vi "Write record log.vi"(4 "Year":i32, 6 "Month":i32, 7 "Instances in":T2[](array[typedef]), 8 "Error In":errorcluster, 11 "refnum":T1) -> (0 "Error Out":errorcluster, 3 "refnum out":T1)   [LabVIEW 2015]
uses:
  Home/Undelivered instance.ctl
  <vilib>/Utility/config.llb/Config Data RefNum.ctl
  <vilib>/Utility/config.llb/Read Key (Path).vi
  <vilib>/Utility/file.llb/Write Delimited Spreadsheet (string).vi
  <vilib>/Utility/config.llb/NI_LVConfig.lvlib
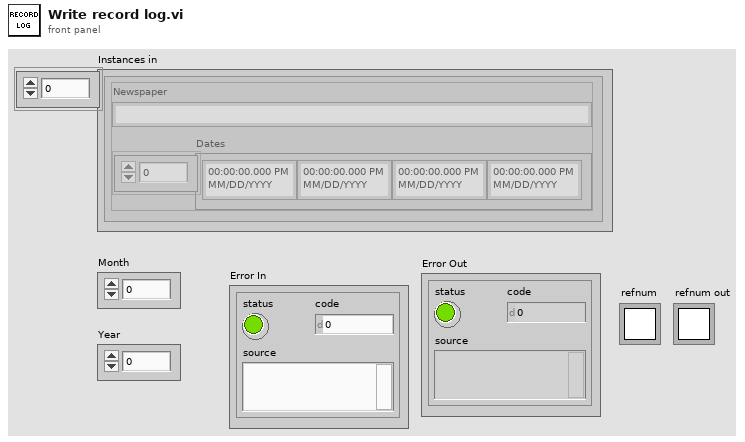
[diagram p1: front panel]
types:
  T1 = typedef "NI_LVConfig.lvlib/Config Data RefNum.ctl" = refnum<k1>
  T2 = typedef "Undelivered instance.ctl" = cluster{"Dates":timestamp[], "Newspaper":string}
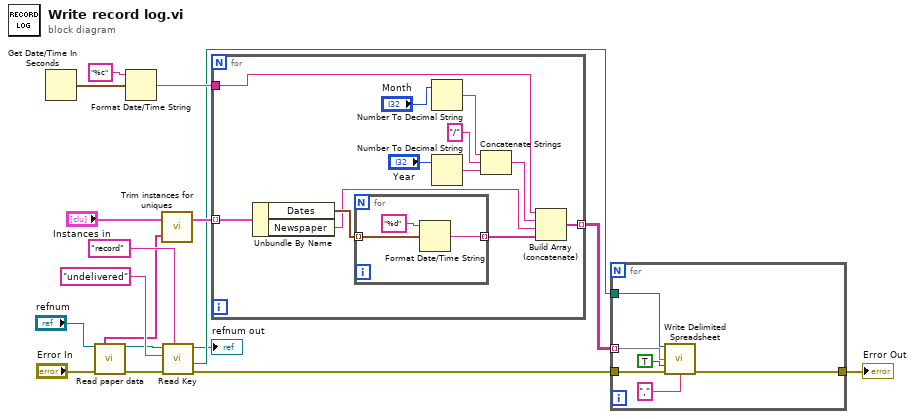
[diagram p0: block diagram]
diagram:
  n1 = Get Date/Time In Seconds() -> (seconds since 1Jan1904=w16:timestamp)
  n2 = call "Read paper data.vi"("Refnum in"="refnum", "error in (no error)"="Error In") -> ("Names"=w1:string[], "Refnum out"=w4:T1, "error out"=w5:errorcluster)  [unwired: 9 in, 2 out]
  n3 = Format Date/Time String(time format string (%c)="%c", seconds (now)=w16) -> (date/time string=w14:string)  [unwired: 1 in]
  n4 = call "Trim instances for uniques.vi"("Paper names"=w1, "Undelivered instances in"="Instances in") -> ("Undelivered instances out"=w17:T2[])
  n5 = call-poly <vilib>:"Read Key.vi"("section"="record", "error in (no error)"=w5, "key"="undelivered", "refnum"=w4) -> ("error out"=w9:errorcluster, "value"=w11:path, "refnum out"=→"refnum out":T1)  [unwired: 4 in, 1 out]
  n6 = for {
    tunnel: w17 -> [w29] mode=indexing
    tunnel: w14 -> [w25]
    tunnel: [w24] -> w10 mode=indexing
    n7 = Unbundle By Name(w29) -> ("Dates"=w28:timestamp[], "Newspaper"=w27:string)
    n8 = for {
      tunnel: w28 -> [w32] mode=indexing
      tunnel: [w30] -> w26 mode=indexing
      n9 = Format Date/Time String(time format string (%c)="%d", seconds (now)=w32) -> (date/time string=w30:string)  [unwired: 1 in]
    }
    n10 = Number To Decimal String(number="Month") -> (decimal integer string=w23:string)  [unwired: 1 in]
    n11 = Number To Decimal String(number="Year") -> (decimal integer string=w21:string)  [unwired: 1 in]
    n12 = Concatenate Strings(w23, "/", w21) -> (w18:string)
    n13 = Build Array (concatenate)(w25, w18, w27, w26) -> (w24:string[])
  }
  n14 = for {
    tunnel: w11 -> [w38]
    tunnel: w10 -> [w36] mode=indexing
    tunnel: w9 -> [w34]
    tunnel: [w33] -> w7
    n15 = call-poly <vilib>:"Write Delimited Spreadsheet.vi"("file path (dialog if empty)"=w38, "1D data"=w36, "append to file? (F)"=TRUE, "error in (no error)"=w34, "delimiter (\\t)"="," ("delimiter (\\t)")) -> ("error out"=w33:errorcluster)  [unwired: 9 in, 1 out]
  }
  "Error Out" <- w7
